vi "HT_multiply_16_2.vi"(8 "input valid":bool=TRUE, 10 "y":fxp<+/-,16,2>, 11 "x":fxp<+/-,16,2>) -> (0 "output valid":bool, 3 "x*y":fxp<+/-,16,2>)   [LabVIEW 2018]
uses:
  <vilib>/rvi/FXPMathLib/FxpConvert/subVIs/nifxpmath_Convert_SimConfig.ctl
  <vilib>/fxp/LVFixedPointQuantizationPolicyTypeDef.ctl
  <vilib>/fxp/LVFixedPointOverflowPolicyTypeDef.ctl
  <vilib>/rvi/FXPMathLib/FxpConvert/simVIs/DllFxpConvertTemp_sub.vi
  <vilib>/rvi/FXPMathLib/FxpConvert/XNode/nifxpmath_Convert.xnode
  <vilib>/rvi/FXPMathLib/FxpMul/XNode/nifxpmath_Multiplier.xnode
  <vilib>/rvi/FXPMathLib/sim/FxpSim.dll
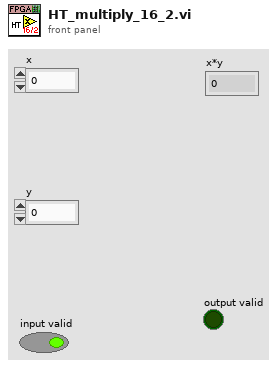
[diagram p1: front panel]
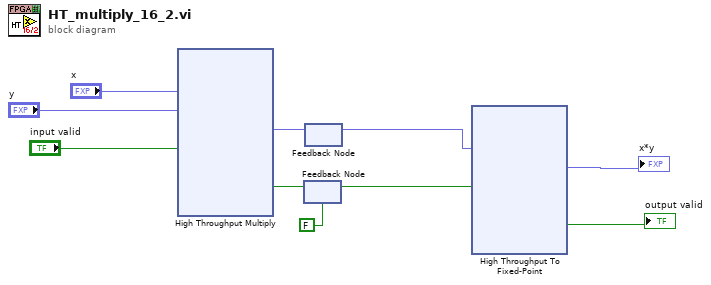
[diagram p0: block diagram]
diagram:
  n1 = xnode ("High Throughput Multiply")("x"="x", "y"="y", "input valid"="input valid") -> ("x*y"=w10:fxp<+/-,32,4>, "output valid"=w9:bool)  [unwired: 1 in, 1 out]
  n2 = feedback #1(FALSE ("output valid")) -> (w4:bool)
  n3 = feedback-in #1(w9) -> ()
  n4 = feedback #2() -> (w1:fxp<+/-,32,4>)  [unwired: 1 in]
  n5 = feedback-in #2(w10) -> ()
  n6 = xnode "High Throughput To Fixed-Point"("x"=w1, "input valid"=w4) -> ("y"=→"x*y":fxp<+/-,16,2>, "output valid"=→"output valid":bool)  [unwired: 1 in, 1 out]
